vi "_Revert CSM Safe String.vi"(11 "Text.Text":string=" \n//Data: Initialize >> http://github.com\n\n\n\nInitialize Core Data  >> http://github.com -> caller\nData: Update Indicators\nInitialize Core Data  >> http://github.com -@ caller\nInitialize Core Data  >> http://github.com ->| caller\nabcd @dasdfa >> asdvev@asdfasdf -><register>") -> (3 "States":string=" \r\n//Data: Initialize >> http://github.com\r\n\r\n\r\n\r\nInitialize Core Data  >> http:%2F%2Fgithub.com\r\nData: Update Indicators")   [LabVIEW 2017]
uses:
  AdvanceAPI/CSM - Keywords.vi
  Communicable State Machine.lvlib
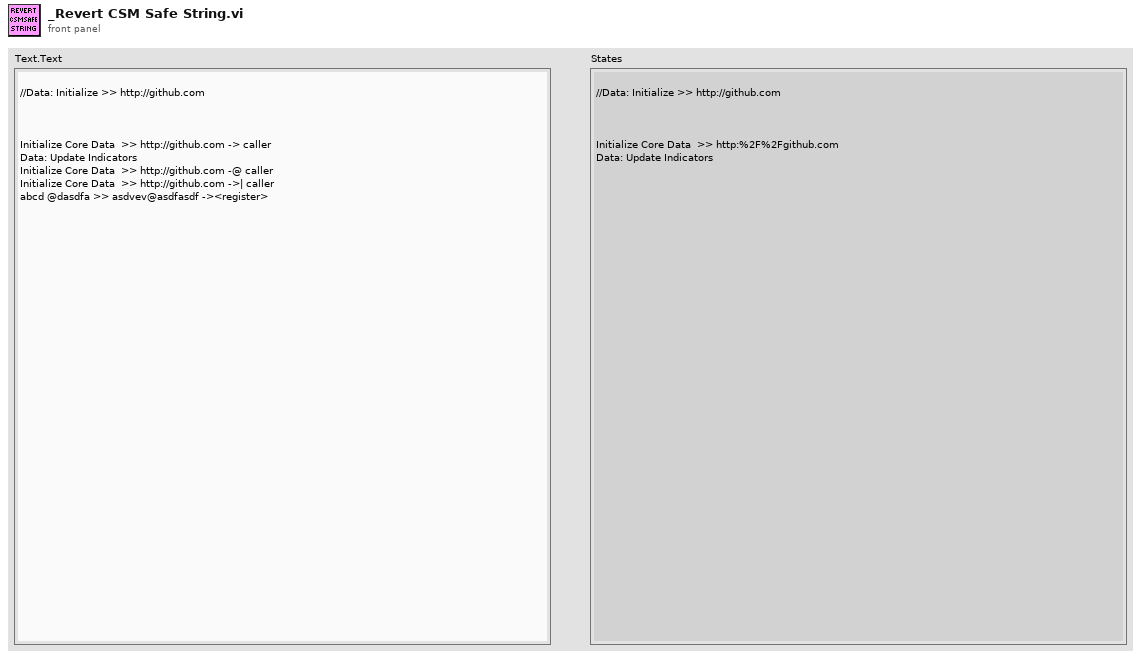
[diagram p1: front panel]
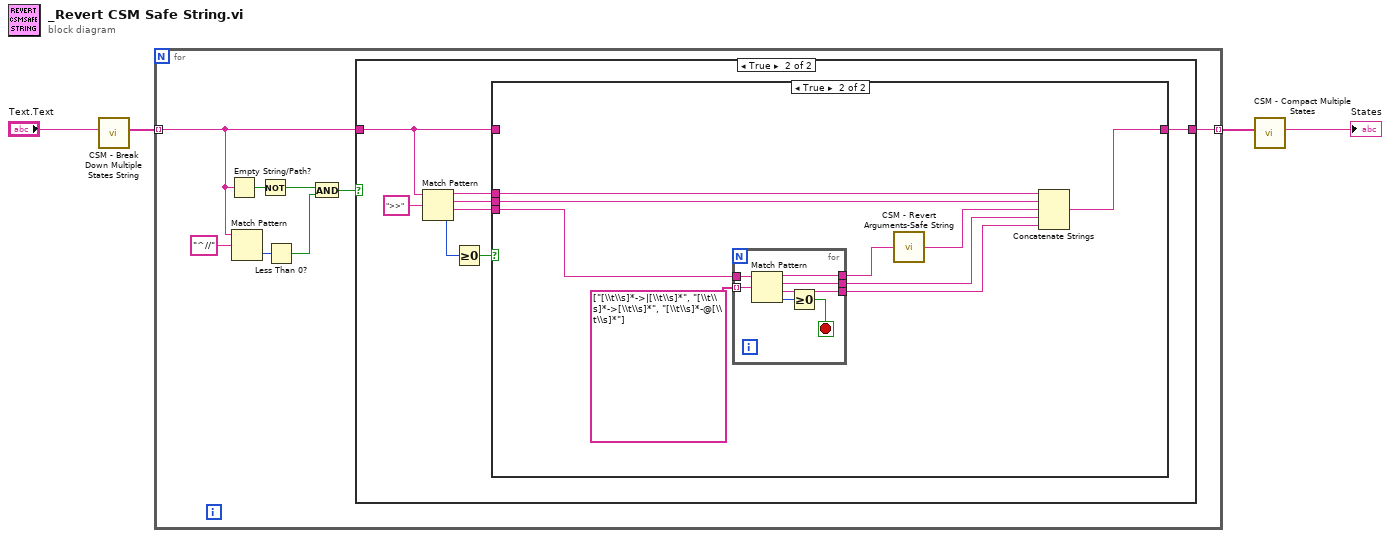
[diagram p0: block diagram]
diagram:
  n1 = call "CSM - Break Down Multiple States String.vi"("States"="Text.Text") -> ("Multiple States"=w3:string[])  [unwired: 10 in]
  n2 = for {
    tunnel: w3 -> [w9] mode=indexing
    tunnel: [w12] -> w4 mode=indexing
    n3 = Empty String/Path?(string/path=w9) -> (empty?=w8:bool)
    n4 = Match Pattern(string=w9, regular expression="^//") -> (offset past match=w11:i32)  [unwired: 1 in, 3 out]
    n5 = Not(x=w8) -> (.not. x?=w7:bool)
    n6 = Less Than 0?(x=w11) -> (x < 0?=w6:bool)
    n7 = And(x=w7, y=w6) -> (x .and. y?=w5:bool)
    n8 = case shown="True" w5 {
      tunnel: [w13 w18] -> w12
      tunnel: w9 -> [w13 w14]
      frame False {
      }
      frame True {
        n9 = Match Pattern(string=w14, regular expression=">>") -> (before substring=w16:string, match substring=w15:string, after substring=w20:string, offset past match=w19:i32)  [unwired: 1 in]
        n10 = Greater Or Equal To 0?(x=w19) -> (x >= 0?=w17:bool)
        n11 = case shown="True" w17 {
          tunnel: w20 -> [_ w31]
          tunnel: [w22 w23] -> w18
          tunnel: w14 -> [w22 _]
          tunnel: w16 -> [_ w28]
          tunnel: w15 -> [_ w27]
          frame False {
          }
          frame True {
            n12 = for {
              tunnel: w31 -> [w38]
              tunnel: string[] ["[\\t\\s]*->|[\\t\\s]*", "[\\t\\s]*->[\\t\\s]*", "[\\t\\s]*-@[\\t\\s]*"] -> [w37] mode=indexing
              tunnel: [w34] -> w30
              tunnel: [w33] -> w25
              tunnel: [w32] -> w24
              stop <- w35 stop-if-true
              n13 = Match Pattern(string=w38, regular expression=w37) -> (before substring=w34:string, match substring=w33:string, after substring=w32:string, offset past match=w36:i32)  [unwired: 1 in]
              n14 = Greater Or Equal To 0?(x=w36) -> (x >= 0?=w35:bool)
            }
            n15 = call "CSM - Revert Arguments-Safe String.vi"("Safe Argument String"=w30) -> ("Origin Argument String"=w26:string)  [unwired: 8 in]
            n16 = Concatenate Strings(w28, w27, w26, w25, w24) -> (w23:string)
          }
        }
      }
    }
  }
  n17 = call "CSM - Compact Multiple States.vi"("Multiple States"=w4) -> ("States"=→"States":string)  [unwired: 9 in]
